vi "Osciloskop.vi"() -> ()   [LabVIEW 2023]
uses:
  <instrlib>/niScope/Controls/niScope scalar measurement.ctl
  <instrlib>/niScope/Utility/niScope Get Channel Name From String.vi
  <instrlib>/niScope/Acquire/Fetch/niScope Fetch WDT.vi
  <vilib>/express/express analysis/Spectral/Block/exnSpectralBlock spectral measurements RMS poly.vi
  <vilib>/express/express analysis/Spectral/Block/exnSpectralBlock spectral measurements RMS DDT.vi
  <vilib>/express/express analysis/Spectral/Block/exnSpectralBlock spectral measurements peak poly.vi
  <vilib>/express/express analysis/Spectral/Block/exnSpectralBlock spectral measurements peak DDT.vi
  <vilib>/express/express analysis/Spectral/Block/exnSpectralBlock spectral measurements power poly.vi
  <vilib>/express/express analysis/Spectral/Block/exnSpectralBlock spectral measurements power DDT.vi
  <vilib>/express/express analysis/Spectral/Block/exnSpectralBlock spectral measurements PSD poly.vi
  <vilib>/express/express analysis/Spectral/Block/exnSpectralBlock spectral measurements PSD DDT.vi
  <vilib>/express/express analysis/Spectral/XNode/ExpressSpectralMeasurementsBlockNode.xnode
panel:
  in  "Resource name":refnum<k15> caption="Device"
  in  "Start/Pause":bool
  in  "Simulation":bool
  in  "Measurement 5":T1=6 caption="Measurement 4" items=["None"=4000, "Frequency"=2, "Average Frequency"=1016, "FFT Frequency"=1008, "Period"=3, "Average Period"=1015, "Rise Time"=0, "Fall Time"=1, "Rising Slew Rate"=1010, "Falling Slew Rate"=1011, "Overshoot"=18, "Preshoot"=19, "Voltage RMS"=4, "Voltage Cycle RMS"=16, "AC Estimate"=1012, "FFT Amplitude"=1009, "Voltage Average"=10, "Voltage Cycle Average"=17, "DC Estimate"=1013, "Voltage Max"=6, "Voltage Min"=7, "Voltage Peak-to-Peak"=5, "Voltage High"=8, "Voltage Low"=9, "Voltage Amplitude"=15, "Voltage Top"=1007, "Voltage Base"=1006, "Voltage Base-to-Top"=1017, "Negative Width"=11, "Positive Width"=12, "Negative Duty Cycle"=13, "Positive Duty Cycle"=14, "Integral"=1005, "Area"=1003, "Cycle Area"=1004, "Time Delay"=1014, "Phase Delay"=1018, "Low Ref Volts"=1000, "Mid Ref Volts"=1001, "High Ref Volts"=1002, "Volt. Hist. Mean"=2000, "Volt. Hist. Stdev"=2001, "Volt. Hist. Median"=2003, "Volt. Hist. Mode"=2010, "Volt. Hist. Max"=2005, "Volt. Hist. Min"=2006, "Volt. Hist. Peak-to-Peak"=2002, "Volt. Hist. Mean + Stdev"=2007, "Volt. Hist. Mean + 2 Stdev"=2008, "Volt. Hist. Mean + 3 Stdev"=2009, "Volt. Hist. Hits"=2004, "Volt. Hist. New Hits"=2011, "Time Hist. Mean"=3000, "Time Hist. Stdev"=3001, "Time Hist. Median"=3003, "Time Hist. Mode"=3010, "Time Hist. Max"=3005, "Time Hist. Min"=3006, "Time Hist. Peak-to-Peak"=3002, "Time Hist. Mean + Stdev"=3007, "Time Hist. Mean + 2 Stdev"=3008, "Time Hist. Mean + 3 Stdev"=3009, "Time Hist. Hits"=3004, "Time Hist. New Hits"=3011]
  in  "Measurement 4":T1=5 caption="Measurement 3" items=["None"=4000, "Frequency"=2, "Average Frequency"=1016, "FFT Frequency"=1008, "Period"=3, "Average Period"=1015, "Rise Time"=0, "Fall Time"=1, "Rising Slew Rate"=1010, "Falling Slew Rate"=1011, "Overshoot"=18, "Preshoot"=19, "Voltage RMS"=4, "Voltage Cycle RMS"=16, "AC Estimate"=1012, "FFT Amplitude"=1009, "Voltage Average"=10, "Voltage Cycle Average"=17, "DC Estimate"=1013, "Voltage Max"=6, "Voltage Min"=7, "Voltage Peak-to-Peak"=5, "Voltage High"=8, "Voltage Low"=9, "Voltage Amplitude"=15, "Voltage Top"=1007, "Voltage Base"=1006, "Voltage Base-to-Top"=1017, "Negative Width"=11, "Positive Width"=12, "Negative Duty Cycle"=13, "Positive Duty Cycle"=14, "Integral"=1005, "Area"=1003, "Cycle Area"=1004, "Time Delay"=1014, "Phase Delay"=1018, "Low Ref Volts"=1000, "Mid Ref Volts"=1001, "High Ref Volts"=1002, "Volt. Hist. Mean"=2000, "Volt. Hist. Stdev"=2001, "Volt. Hist. Median"=2003, "Volt. Hist. Mode"=2010, "Volt. Hist. Max"=2005, "Volt. Hist. Min"=2006, "Volt. Hist. Peak-to-Peak"=2002, "Volt. Hist. Mean + Stdev"=2007, "Volt. Hist. Mean + 2 Stdev"=2008, "Volt. Hist. Mean + 3 Stdev"=2009, "Volt. Hist. Hits"=2004, "Volt. Hist. New Hits"=2011, "Time Hist. Mean"=3000, "Time Hist. Stdev"=3001, "Time Hist. Median"=3003, "Time Hist. Mode"=3010, "Time Hist. Max"=3005, "Time Hist. Min"=3006, "Time Hist. Peak-to-Peak"=3002, "Time Hist. Mean + Stdev"=3007, "Time Hist. Mean + 2 Stdev"=3008, "Time Hist. Mean + 3 Stdev"=3009, "Time Hist. Hits"=3004, "Time Hist. New Hits"=3011]
  in  "Measurement 3":T1 caption="Measurement 2" items=["None"=4000, "Frequency"=2, "Average Frequency"=1016, "FFT Frequency"=1008, "Period"=3, "Average Period"=1015, "Rise Time"=0, "Fall Time"=1, "Rising Slew Rate"=1010, "Falling Slew Rate"=1011, "Overshoot"=18, "Preshoot"=19, "Voltage RMS"=4, "Voltage Cycle RMS"=16, "AC Estimate"=1012, "FFT Amplitude"=1009, "Voltage Average"=10, "Voltage Cycle Average"=17, "DC Estimate"=1013, "Voltage Max"=6, "Voltage Min"=7, "Voltage Peak-to-Peak"=5, "Voltage High"=8, "Voltage Low"=9, "Voltage Amplitude"=15, "Voltage Top"=1007, "Voltage Base"=1006, "Voltage Base-to-Top"=1017, "Negative Width"=11, "Positive Width"=12, "Negative Duty Cycle"=13, "Positive Duty Cycle"=14, "Integral"=1005, "Area"=1003, "Cycle Area"=1004, "Time Delay"=1014, "Phase Delay"=1018, "Low Ref Volts"=1000, "Mid Ref Volts"=1001, "High Ref Volts"=1002, "Volt. Hist. Mean"=2000, "Volt. Hist. Stdev"=2001, "Volt. Hist. Median"=2003, "Volt. Hist. Mode"=2010, "Volt. Hist. Max"=2005, "Volt. Hist. Min"=2006, "Volt. Hist. Peak-to-Peak"=2002, "Volt. Hist. Mean + Stdev"=2007, "Volt. Hist. Mean + 2 Stdev"=2008, "Volt. Hist. Mean + 3 Stdev"=2009, "Volt. Hist. Hits"=2004, "Volt. Hist. New Hits"=2011, "Time Hist. Mean"=3000, "Time Hist. Stdev"=3001, "Time Hist. Median"=3003, "Time Hist. Mode"=3010, "Time Hist. Max"=3005, "Time Hist. Min"=3006, "Time Hist. Peak-to-Peak"=3002, "Time Hist. Mean + Stdev"=3007, "Time Hist. Mean + 2 Stdev"=3008, "Time Hist. Mean + 3 Stdev"=3009, "Time Hist. Hits"=3004, "Time Hist. New Hits"=3011]
  in  "Measurement 2":T1=2 caption="Measurement 1" items=["None"=4000, "Frequency"=2, "Average Frequency"=1016, "FFT Frequency"=1008, "Period"=3, "Average Period"=1015, "Rise Time"=0, "Fall Time"=1, "Rising Slew Rate"=1010, "Falling Slew Rate"=1011, "Overshoot"=18, "Preshoot"=19, "Voltage RMS"=4, "Voltage Cycle RMS"=16, "AC Estimate"=1012, "FFT Amplitude"=1009, "Voltage Average"=10, "Voltage Cycle Average"=17, "DC Estimate"=1013, "Voltage Max"=6, "Voltage Min"=7, "Voltage Peak-to-Peak"=5, "Voltage High"=8, "Voltage Low"=9, "Voltage Amplitude"=15, "Voltage Top"=1007, "Voltage Base"=1006, "Voltage Base-to-Top"=1017, "Negative Width"=11, "Positive Width"=12, "Negative Duty Cycle"=13, "Positive Duty Cycle"=14, "Integral"=1005, "Area"=1003, "Cycle Area"=1004, "Time Delay"=1014, "Phase Delay"=1018, "Low Ref Volts"=1000, "Mid Ref Volts"=1001, "High Ref Volts"=1002, "Volt. Hist. Mean"=2000, "Volt. Hist. Stdev"=2001, "Volt. Hist. Median"=2003, "Volt. Hist. Mode"=2010, "Volt. Hist. Max"=2005, "Volt. Hist. Min"=2006, "Volt. Hist. Peak-to-Peak"=2002, "Volt. Hist. Mean + Stdev"=2007, "Volt. Hist. Mean + 2 Stdev"=2008, "Volt. Hist. Mean + 3 Stdev"=2009, "Volt. Hist. Hits"=2004, "Volt. Hist. New Hits"=2011, "Time Hist. Mean"=3000, "Time Hist. Stdev"=3001, "Time Hist. Median"=3003, "Time Hist. Mode"=3010, "Time Hist. Max"=3005, "Time Hist. Min"=3006, "Time Hist. Peak-to-Peak"=3002, "Time Hist. Mean + Stdev"=3007, "Time Hist. Mean + 2 Stdev"=3008, "Time Hist. Mean + 3 Stdev"=3009, "Time Hist. Hits"=3004, "Time Hist. New Hits"=3011]
  in  "Selected Measurement":u16(ring) items=["Magnitude(RMS)", "Magnitude(Peak)", "Power spectrum", "Power spectral density"]
  in  "Left/Right":dbl(knob) scale=-100.0..100.0
  in  "Amp":dbl=1.0 min=1.0 max=1000.0
  in  "Averaging":u16(ring) items=["None", "RMS", "Peak hold"]
  in  "Window":u16(ring) items=["None", "Hanning", "Hamming", "Blackman-Harris", "Exact Blackman", "Blackman", "Flat Top", "4 Term B-Harris", "7 Term B-Harris", "Low Sidelobe"]
  in  "FFT":bool
  out "FFT Graph":dynamicdata(graph)
  in  "Upper Cut-Off":dbl=10.0 caption="Lower Cut-Off"
  in  "Zoom H":dbl(knob)=1.0 scale=0.0..10.0
  in  "Zoom V":dbl(knob)=1.0 scale=0.0..10.0
  in  "Filter":u16(ring) items=["No filter", "Low pass", "High pass", "Band pass", "Band reject", "Smoothing"]
  in  "Lower Cut-Off":dbl=0.5
  in  "Down/Up":dbl(knob) scale=-100.0..100.0
  out "M5":dbl caption="Result  4" format="%.2f"
  out "M4":dbl caption="Result  3" format="%.2f"
  out "M3":dbl caption="Result  2" format="%.2f"
  out "M2":dbl caption="Result 1" format="%.2f"
  in  "Channel/s":string="0"
  out "Waveform Graph":waveform(dbl)[](graph)
  in  "?":bool
  # "Vertical"
  # "Horizontal"
  # "Measuring"
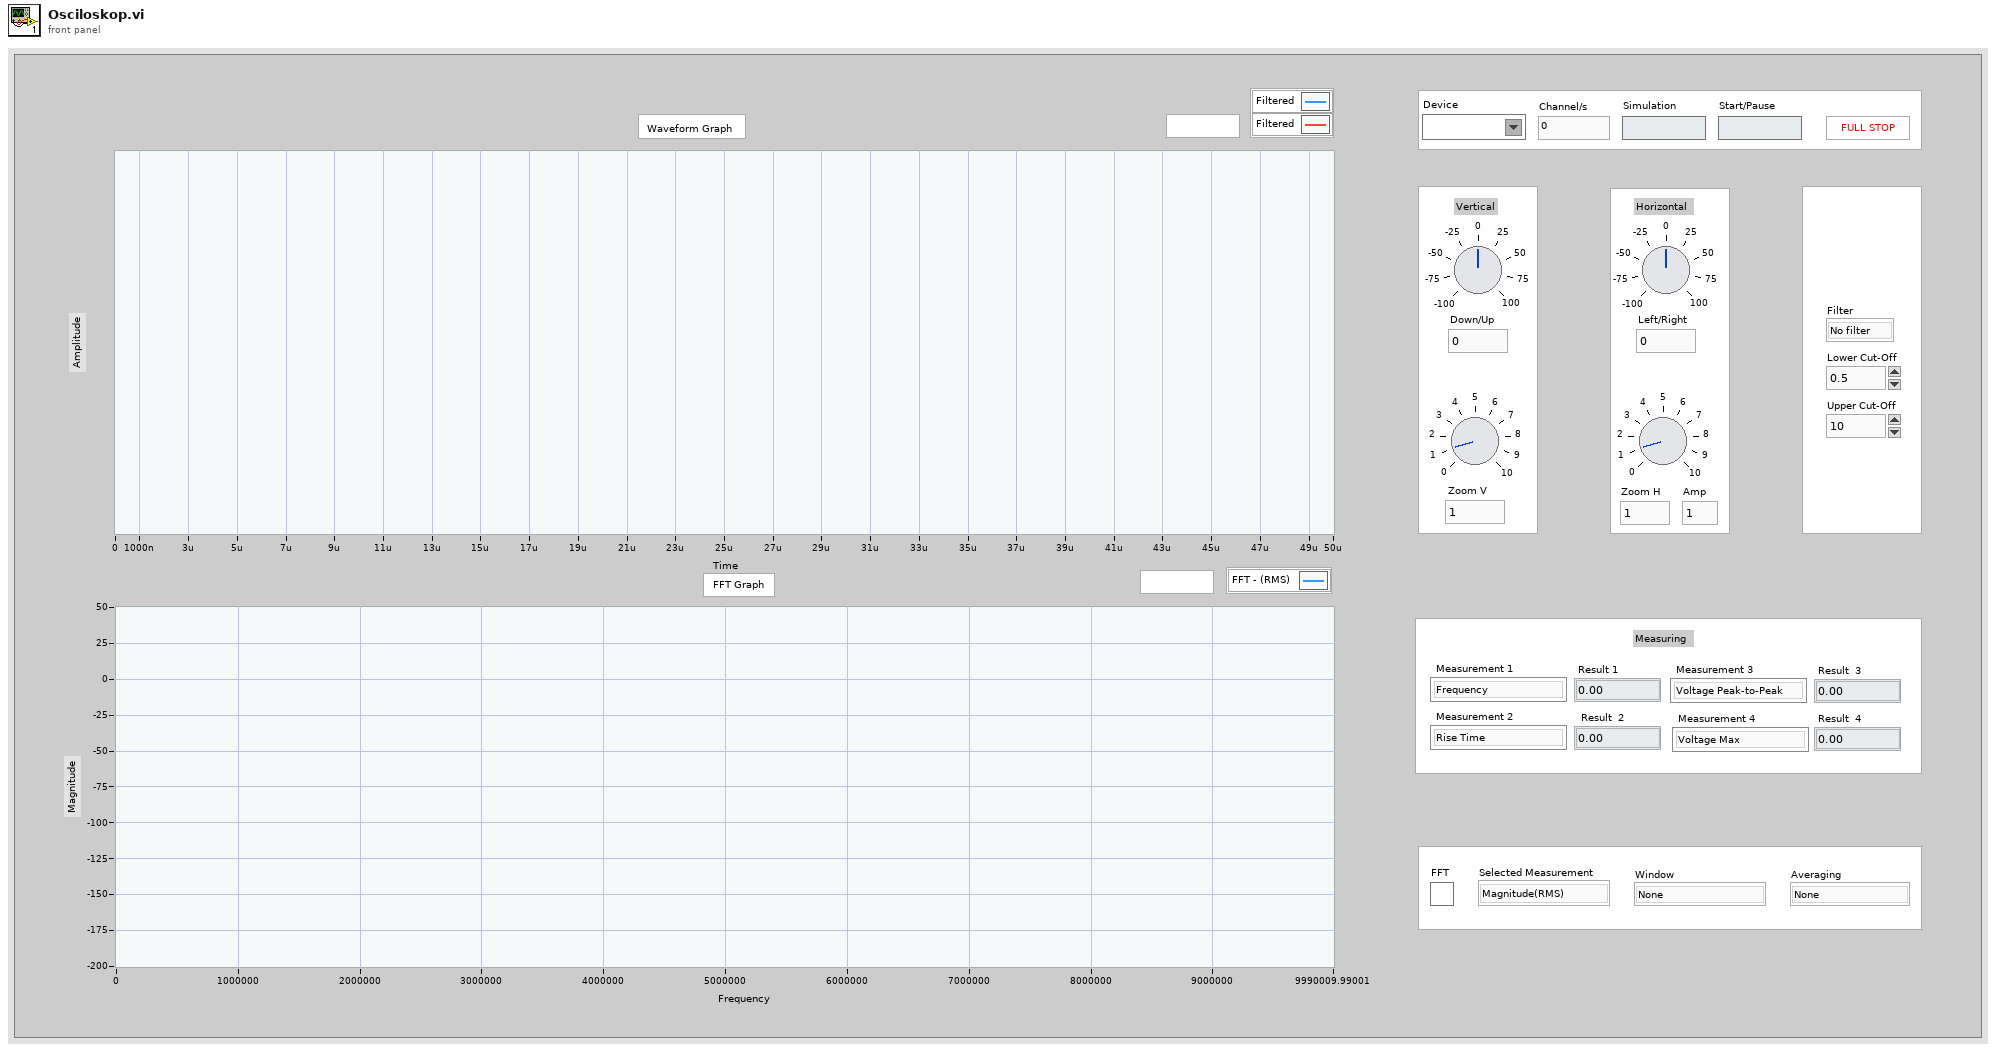
[diagram p1: front panel]
types:
  T1 = typedef "niScope scalar measurement.ctl" = i32
  T2 = cluster{"averaging mode":u16, "weighting mode":u16, "number of averages":u32}
  T3 = cluster{"dB On (F)":bool, "unwrap phase (F)":bool, "convert to degree (F)":bool}
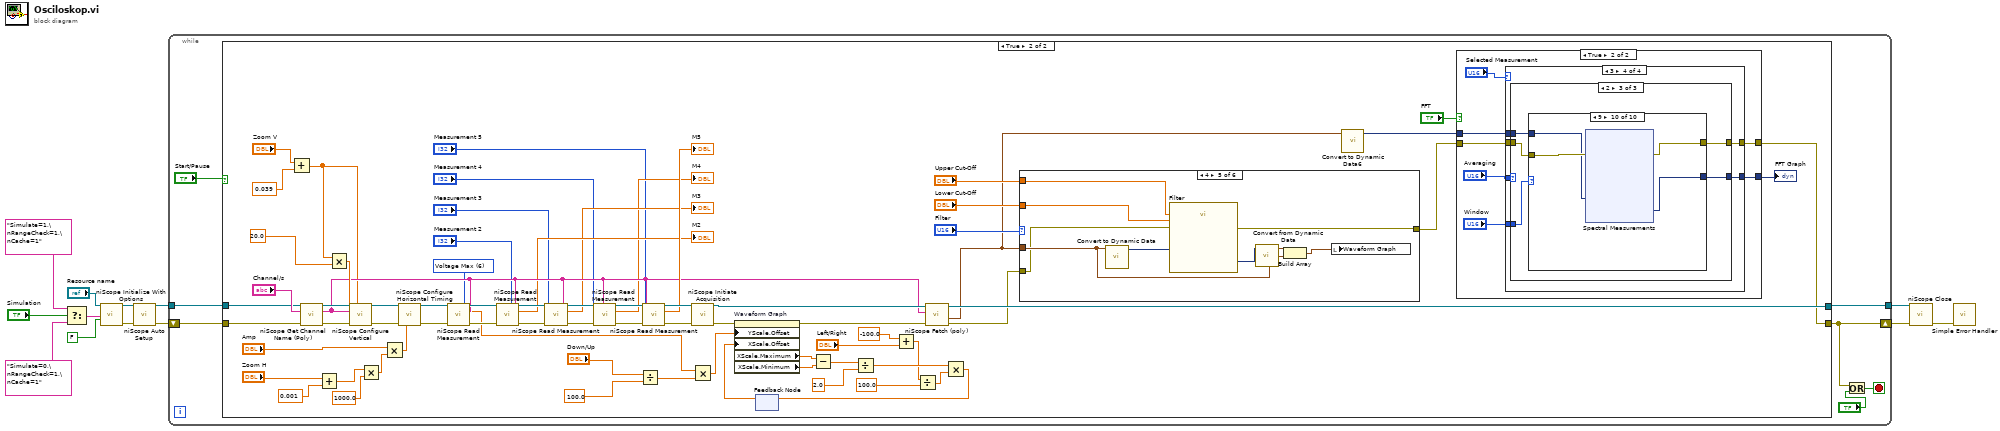
[diagram p0: block diagram]
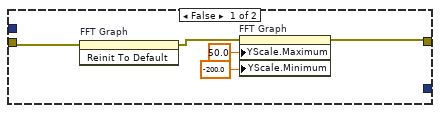
[diagram p3: hidden frame]
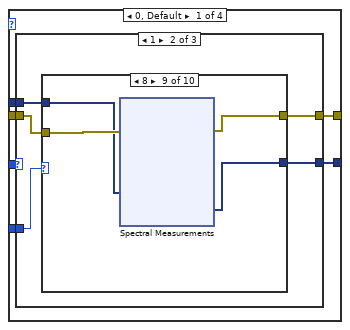
[diagram p4: hidden frame]
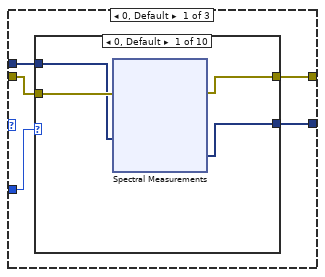
[diagram p5: hidden frame]
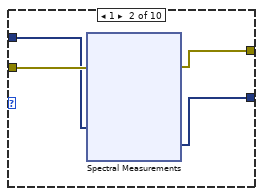
[diagram p6: hidden frame]
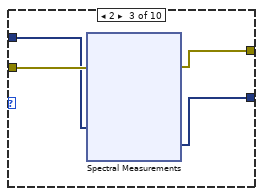
[diagram p7: hidden frame]
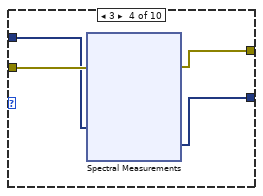
[diagram p8: hidden frame]
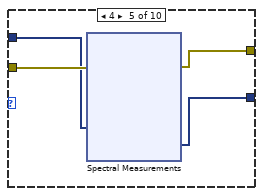
[diagram p9: hidden frame]
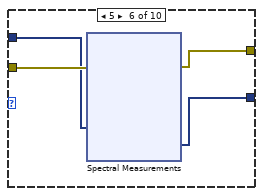
[diagram p10: hidden frame]
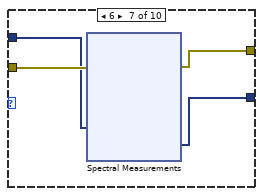
[diagram p11: hidden frame]
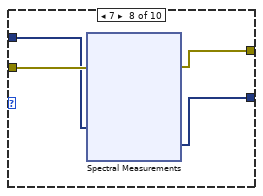
[diagram p12: hidden frame]
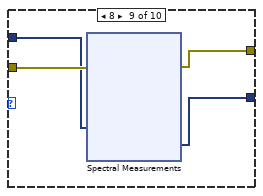
[diagram p13: hidden frame]
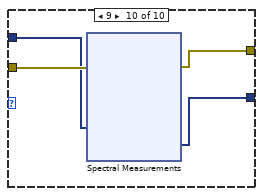
[diagram p14: hidden frame]
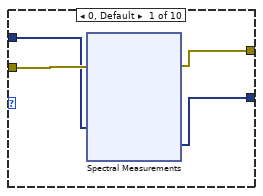
[diagram p15: hidden frame]
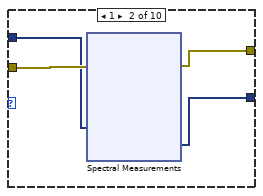
[diagram p16: hidden frame]
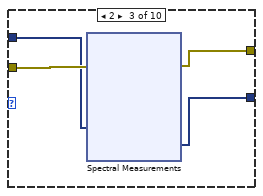
[diagram p17: hidden frame]
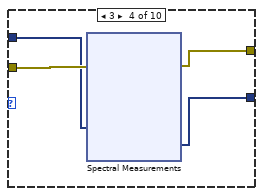
[diagram p18: hidden frame]
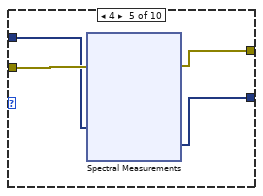
[diagram p19: hidden frame]
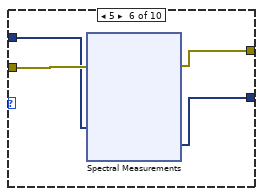
[diagram p20: hidden frame]
diagram:
  n1 = Select(t="Simulate=1,\nRangeCheck=1,\nCache=1" ("option string"), s="Simulation", f="Simulate=0,\nRangeCheck=1,\nCache=1" ("option string")) -> (s? t:f=w9:string)
  n2 = call <instrlib>:"niScope Initialize With Options.vi"("resource name"="Resource name", "option string"=w9, "reset device"=FALSE) -> ("instrument handle"=w7:refnum<k15>, "error out"=w8:errorcluster)  [unwired: 11 in]
  n3 = call <instrlib>:"niScope Auto Setup.vi"("instrument handle"=w7, "error in"=w8) -> ("instrument handle out"=w6:refnum<k15>, "error out"=w4:errorcluster)  [unwired: 12 in]
  n4 = while {
    tunnel: w6 -> [w18]
    shift-right: [w15] -> w5
    shift-left: w4 -> [w17]
    tunnel: [w16] -> w3
    stop <- w19 stop-if-true
    n5 = case shown="True" "Start/Pause" {
      tunnel: [w21 w91] -> w16
      tunnel: w17 -> [w22 w58]
      tunnel: w18 -> [w21 w57]
      tunnel: [w22 w56] -> w15
      frame False {
      }
      frame True {
        w26 = T1 6 items=["None"=4000, "Frequency"=2, "Average Frequency"=1016, "FFT Frequency"=1008, "Period"=3, "Average Period"=1015, "Rise Time"=0, "Fall Time"=1, "Rising Slew Rate"=1010, "Falling Slew Rate"=1011, "Overshoot"=18, "Preshoot"=19, "Voltage RMS"=4, "Voltage Cycle RMS"=16, "AC Estimate"=1012, "FFT Amplitude"=1009, "Voltage Average"=10, "Voltage Cycle Average"=17, "DC Estimate"=1013, "Voltage Max"=6, "Voltage Min"=7, "Voltage Peak-to-Peak"=5, "Voltage High"=8, "Voltage Low"=9, "Voltage Amplitude"=15, "Voltage Top"=1007, "Voltage Base"=1006, "Voltage Base-to-Top"=1017, "Negative Width"=11, "Positive Width"=12, "Negative Duty Cycle"=13, "Positive Duty Cycle"=14, "Integral"=1005, "Area"=1003, "Cycle Area"=1004, "Time Delay"=1014, "Phase Delay"=1018, "Low Ref Volts"=1000, "Mid Ref Volts"=1001, "High Ref Volts"=1002, "Volt. Hist. Mean"=2000, "Volt. Hist. Stdev"=2001, "Volt. Hist. Median"=2003, "Volt. Hist. Mode"=2010, "Volt. Hist. Max"=2005, "Volt. Hist. Min"=2006, "Volt. Hist. Peak-to-Peak"=2002, "Volt. Hist. Mean + Stdev"=2007, "Volt. Hist. Mean + 2 Stdev"=2008, "Volt. Hist. Mean + 3 Stdev"=2009, "Volt. Hist. Hits"=2004, "Volt. Hist. New Hits"=2011, "Time Hist. Mean"=3000, "Time Hist. Stdev"=3001, "Time Hist. Median"=3003, "Time Hist. Mode"=3010, "Time Hist. Max"=3005, "Time Hist. Min"=3006, "Time Hist. Peak-to-Peak"=3002, "Time Hist. Mean + Stdev"=3007, "Time Hist. Mean + 2 Stdev"=3008, "Time Hist. Mean + 3 Stdev"=3009, "Time Hist. Hits"=3004, "Time Hist. New Hits"=3011] ("scalar measurement")
        n6 = Add(x="Zoom V", y=0.039) -> (x+y=w23:dbl)
        n7 = call-poly <instrlib>:"niScope Get Channel Name (Poly).vi"("instrument handle"=w57, "index"="Channel/s", "error in"=w58) -> ("instrument handle out"=w94:refnum<k15>, "channel name"=w53:string, "error out"=w93:errorcluster)  [unwired: 10 in]
        n8 = Add(x="Zoom H", y=0.001) -> (x+y=w44:dbl)
        n9 = Multiply(x=w23, y=20.0) -> (x*y=w84:dbl)
        n10 = call <instrlib>:"niScope Configure Vertical.vi"("instrument handle"=w94, "probe attenuation"=w23, "channels"=w53, "vertical range"=w84, "error in"=w93) -> ("instrument handle out"=w24:refnum<k15>, "error out"=w25:errorcluster)  [unwired: 9 in]
        n11 = Multiply(x=w44, y=1000.0 ("x")) -> (x*y=w43:dbl)
        n12 = Multiply(x="Amp", y=w43) -> (x*y=w83:dbl)
        n13 = call <instrlib>:"niScope Configure Horizontal Timing.vi"("instrument handle"=w24, "error in"=w25, "min record length"=w83) -> ("instrument handle out"=w77:refnum<k15>, "error out"=w78:errorcluster)  [unwired: 11 in]
        n14 = call <instrlib>:"niScope Read Measurement.vi"("instrument handle"=w77, "channels"=w53, "scalar measurement"=w26, "error in"=w78) -> ("instrument handle out"=w68:refnum<k15>, "result"=w52:dbl, "error out"=w63:errorcluster)  [unwired: 9 in]
        n15 = call <instrlib>:"niScope Read Measurement.vi"("instrument handle"=w68, "channels"=w53, "scalar measurement"="Measurement 2", "error in"=w63) -> ("instrument handle out"=w67:refnum<k15>, "result"=→"M2":dbl, "error out"=w62:errorcluster)  [unwired: 9 in]
        n16 = call <instrlib>:"niScope Read Measurement.vi"("instrument handle"=w67, "channels"=w53, "scalar measurement"="Measurement 3", "error in"=w62) -> ("instrument handle out"=w66:refnum<k15>, "result"=→"M3":dbl, "error out"=w61:errorcluster)  [unwired: 9 in]
        n17 = call <instrlib>:"niScope Read Measurement.vi"("instrument handle"=w66, "channels"=w53, "scalar measurement"="Measurement 4", "error in"=w61) -> ("instrument handle out"=w65:refnum<k15>, "result"=→"M4":dbl, "error out"=w60:errorcluster)  [unwired: 9 in]
        n18 = Divide(x="Down/Up", y=100.0) -> (x/y=w38:dbl)
        n19 = call <instrlib>:"niScope Read Measurement.vi"("instrument handle"=w65, "channels"=w53, "scalar measurement"="Measurement 5", "error in"=w60) -> ("instrument handle out"=w64:refnum<k15>, "result"=→"M5":dbl, "error out"=w59:errorcluster)  [unwired: 9 in]
        n20 = call <instrlib>:"niScope Initiate Acquisition.vi"("instrument handle"=w64, "error in"=w59) -> ("instrument handle out"=w80:refnum<k15>, "error out"=w79:errorcluster)  [unwired: 12 in]
        n21 = Multiply(x=w52, y=w38) -> (x*y=w76:dbl)
        n22 = feedback #1() -> (w71:dbl)  [unwired: 1 in]
        n23 = property on="Waveform Graph" class="WFGraph (strict)"(error in=w79, "YScale.Offset"=w76, "XScale.Offset"=w71) -> (error out=w82:errorcluster, "XScale.Maximum"=w36:dbl, "XScale.Minimum"=w35:dbl)  [unwired: 1 in, 1 out]
        n24 = Subtract(x=w36, y=w35) -> (x-y=w75:dbl)
        n25 = Divide(x=w75, y=2.0) -> (x/y=w73:dbl)
        n26 = Add(x=-100.0, y="Left/Right") -> (x+y=w33:dbl)
        n27 = Divide(x=w33, y=100.0) -> (x/y=w32:dbl)
        n28 = call-poly <instrlib>:"niScope Fetch (poly).vi"("error in"=w82, "channels"=w53, "instrument handle"=w80) -> ("error out"=w27:errorcluster, "wfm"=w28:waveform(dbl), "instrument handle out"=w91:refnum<k15>)  [unwired: 5 in, 1 out]
        n29 = Multiply(x=w73, y=w32) -> (x*y=w72:dbl)
        n30 = feedback-in #1(w72) -> ()
        n31 = case shown="4" "Filter" {
          tunnel: "Lower Cut-Off" -> [_ w1900 w1908 w1918 w1927 _]
          tunnel: w28 -> [w1893 w1897 w1905 w1914 w1923 w1932]
          tunnel: "Upper Cut-Off" -> [_ _ _ w1912 w1921 _]
          tunnel: w27 -> [w1891 w1895 w1903 w1910 w1920 w1928]
          tunnel: [w1891 w1894 w1902 w1911 w1919 w1929] -> w55
          frame 0, Default {
            n32 = Build Array(w1893, w1893) -> (→"Waveform Graph":waveform(dbl)[])
          }
          frame 1 {
            n33 = call "Convert to Dynamic Data2"("Waveform"=w1897) -> ("Dynamic Data Type"=w1899:dynamicdata)  [unwired: 3 in]
            n34 = call "Filter2"("error in (no error)"=w1895, "Lower Cut-Off"=w1900, "Signal"=w1899) -> ("error out"=w1894:errorcluster, "Filtered Signal"=w1901:dynamicdata)  [unwired: 7 in]
            n35 = call "Convert from Dynamic Data2"("Dynamic Data Type"=w1901) -> ("Waveform"=w1898:waveform(dbl))  [unwired: 3 in]
            n36 = Build Array(w1898, w1897) -> (w1896:waveform(dbl)[])
            n37 = local write "Waveform Graph"(w1896) -> ()
          }
          frame 2 {
            n38 = call "Convert to Dynamic Data3"("Waveform"=w1905) -> ("Dynamic Data Type"=w1907:dynamicdata)  [unwired: 3 in]
            n39 = call "Filter3"("error in (no error)"=w1903, "Lower Cut-Off"=w1908, "Signal"=w1907) -> ("error out"=w1902:errorcluster, "Filtered Signal"=w1909:dynamicdata)  [unwired: 7 in]
            n40 = call "Convert from Dynamic Data3"("Dynamic Data Type"=w1909) -> ("Waveform"=w1906:waveform(dbl))  [unwired: 3 in]
            n41 = Build Array(w1906, w1905) -> (w1904:waveform(dbl)[])
            n42 = local write "Waveform Graph"(w1904) -> ()
          }
          frame 3 {
            n43 = call "Convert to Dynamic Data4"("Waveform"=w1914) -> ("Dynamic Data Type"=w1917:dynamicdata)  [unwired: 3 in]
            n44 = call "Filter4"("error in (no error)"=w1910, "Lower Cut-Off"=w1918, "Upper Cut-Off"=w1912, "Signal"=w1917) -> ("error out"=w1911:errorcluster, "Filtered Signal"=w1916:dynamicdata)  [unwired: 6 in]
            n45 = call "Convert from Dynamic Data4"("Dynamic Data Type"=w1916, "Channel"=w1916) -> ("Waveform"=w1915:waveform(dbl))  [unwired: 2 in]
            n46 = Build Array(w1915, w1914) -> (w1913:waveform(dbl)[])
            n47 = local write "Waveform Graph"(w1913) -> ()
          }
          frame 4 {
            n48 = call "Convert to Dynamic Data"("Waveform"=w1923) -> ("Dynamic Data Type"=w1926:dynamicdata)  [unwired: 3 in]
            n49 = call "Filter"("error in (no error)"=w1920, "Lower Cut-Off"=w1927, "Upper Cut-Off"=w1921, "Signal"=w1926) -> ("error out"=w1919:errorcluster, "Filtered Signal"=w1925:dynamicdata)  [unwired: 6 in]
            n50 = call "Convert from Dynamic Data"("Dynamic Data Type"=w1925, "Channel"=w1925) -> ("Waveform"=w1924:waveform(dbl))  [unwired: 2 in]
            n51 = Build Array(w1924, w1923) -> (w1922:waveform(dbl)[])
            n52 = local write "Waveform Graph"(w1922) -> ()
          }
          frame 5 {
            n53 = call "Convert to Dynamic Data5"("Waveform"=w1932) -> ("Dynamic Data Type"=w1934:dynamicdata)  [unwired: 3 in]
            n54 = call "Filter5"("error in (no error)"=w1928, "Signal"=w1934) -> ("error out"=w1929:errorcluster, "Filtered Signal"=w1933:dynamicdata)  [unwired: 8 in]
            n55 = call "Convert from Dynamic Data5"("Dynamic Data Type"=w1933, "Channel"=w1933) -> ("Waveform"=w1930:waveform(dbl))  [unwired: 2 in]
            n56 = Build Array(w1930, w1930) -> (w1931:waveform(dbl)[])
            n57 = local write "Waveform Graph"(w1931) -> ()
          }
        }
        n58 = call "Convert to Dynamic Data6"("Waveform"=w28) -> ("Dynamic Data Type"=w86:dynamicdata)  [unwired: 3 in]
        n59 = case shown="True" "FFT" {
          tunnel: w55 -> [w99 w104]
          tunnel: [w97 w102] -> w56
          tunnel: w86 -> [_ w103]
          tunnel: [_ w100] -> w85
          frame False {
            n60 = invoke on="FFT Graph" class="WFGraph (strict)" method="Reinit To Default"(error in=w99) -> (error out=w98:errorcluster)  [unwired: 2 in, 2 out]
            n61 = property on="FFT Graph" class="WFGraph (strict)"(error in=w98, "YScale.Maximum"=50.0 ("Y Scale.Range:Maximum"), "YScale.Minimum"=-200.0 ("Y Scale.Range:Minimum")) -> (error out=w97:errorcluster)  [unwired: 1 in, 1 out]
          }
          frame True {
            n62 = case shown="3" "Selected Measurement" {
              tunnel: "Averaging" -> [w112 w573 w1034 w1465]
              tunnel: "Window" -> [w111 w572 w1033 w1464]
              tunnel: w104 -> [w110 w571 w1032 w1463]
              tunnel: w103 -> [w109 w570 w1031 w1462]
              tunnel: [w108 w569 w1030 w1461] -> w102
              tunnel: [w107 w568 w1029 w1460] -> w100
              frame 0, Default {
                n63 = case shown="1" w112 {
                  tunnel: w111 -> [w117 w262 w417]
                  tunnel: w110 -> [w116 w261 w416]
                  tunnel: w109 -> [w115 w260 w415]
                  tunnel: [w114 w259 w414] -> w108
                  tunnel: [w113 w258 w413] -> w107
                  frame 0, Default {
                    n64 = case shown="0, Default" w117 {
                      tunnel: w116 -> [w121 w135 w149 w163 w177 w191 w205 w219 w233 w247]
                      tunnel: w115 -> [w120 w134 w148 w162 w176 w190 w204 w218 w232 w246]
                      tunnel: [w119 w133 w147 w161 w175 w189 w203 w217 w231 w245] -> w114
                      tunnel: [w118 w132 w146 w160 w174 w188 w202 w216 w230 w244] -> w113
                      frame 0, Default {
                        n65 = xnode "Spectral Measurements"("Signals"=w120, "error in (no error)"=w121) -> ("FFT - (RMS)"=w118:dynamicdata, "error out"=w119:errorcluster)  [unwired: 1 out]
                      }
                      frame 1 {
                        n66 = xnode "Spectral Measurements"("Signals"=w134, "error in (no error)"=w135) -> ("FFT - (RMS)"=w132:dynamicdata, "error out"=w133:errorcluster)  [unwired: 1 out]
                      }
                      frame 2 {
                        n67 = xnode "Spectral Measurements"("Signals"=w148, "error in (no error)"=w149) -> ("FFT - (RMS)"=w146:dynamicdata, "error out"=w147:errorcluster)  [unwired: 1 out]
                      }
                      frame 3 {
                        n68 = xnode "Spectral Measurements"("Signals"=w162, "error in (no error)"=w163) -> ("FFT - (RMS)"=w160:dynamicdata, "error out"=w161:errorcluster)  [unwired: 1 out]
                      }
                      frame 4 {
                        n69 = xnode "Spectral Measurements"("Signals"=w176, "error in (no error)"=w177) -> ("FFT - (RMS)"=w174:dynamicdata, "error out"=w175:errorcluster)  [unwired: 1 out]
                      }
                      frame 5 {
                        n70 = xnode "Spectral Measurements"("Signals"=w190, "error in (no error)"=w191) -> ("FFT - (RMS)"=w188:dynamicdata, "error out"=w189:errorcluster)  [unwired: 1 out]
                      }
                      frame 6 {
                        n71 = xnode "Spectral Measurements"("Signals"=w204, "error in (no error)"=w205) -> ("FFT - (RMS)"=w202:dynamicdata, "error out"=w203:errorcluster)  [unwired: 1 out]
                      }
                      frame 7 {
                        n72 = xnode "Spectral Measurements"("Signals"=w218, "error in (no error)"=w219) -> ("FFT - (RMS)"=w216:dynamicdata, "error out"=w217:errorcluster)  [unwired: 1 out]
                      }
                      frame 8 {
                        n73 = xnode "Spectral Measurements"("Signals"=w232, "error in (no error)"=w233) -> ("FFT - (RMS)"=w230:dynamicdata, "error out"=w231:errorcluster)  [unwired: 1 out]
                      }
                      frame 9 {
                        n74 = xnode "Spectral Measurements"("Signals"=w246, "error in (no error)"=w247) -> ("FFT - (RMS)"=w244:dynamicdata, "error out"=w245:errorcluster)  [unwired: 1 out]
                      }
                    }
                  }
                  frame 1 {
                    n75 = case shown="8" w262 {
                      tunnel: w261 -> [w266 w281 w296 w311 w326 w341 w356 w371 w386 w401]
                      tunnel: w260 -> [w265 w280 w295 w310 w325 w340 w355 w370 w385 w400]
                      tunnel: [w264 w279 w294 w309 w324 w339 w354 w369 w384 w399] -> w259
                      tunnel: [w263 w278 w293 w308 w323 w338 w353 w368 w383 w398] -> w258
                      frame 0, Default {
                        n76 = xnode "Spectral Measurements"("Signals"=w265, "error in (no error)"=w266) -> ("FFT - (RMS)"=w263:dynamicdata, "error out"=w264:errorcluster)  [unwired: 1 in, 2 out]
                      }
                      frame 1 {
                        n77 = xnode "Spectral Measurements"("Signals"=w280, "error in (no error)"=w281) -> ("FFT - (RMS)"=w278:dynamicdata, "error out"=w279:errorcluster)  [unwired: 1 in, 2 out]
                      }
                      frame 2 {
                        n78 = xnode "Spectral Measurements"("Signals"=w295, "error in (no error)"=w296) -> ("FFT - (RMS)"=w293:dynamicdata, "error out"=w294:errorcluster)  [unwired: 1 in, 2 out]
                      }
                      frame 3 {
                        n79 = xnode "Spectral Measurements"("Signals"=w310, "error in (no error)"=w311) -> ("FFT - (RMS)"=w308:dynamicdata, "error out"=w309:errorcluster)  [unwired: 1 in, 2 out]
                      }
                      frame 4 {
                        n80 = xnode "Spectral Measurements"("Signals"=w325, "error in (no error)"=w326) -> ("FFT - (RMS)"=w323:dynamicdata, "error out"=w324:errorcluster)  [unwired: 1 in, 2 out]
                      }
                      frame 5 {
                        n81 = xnode "Spectral Measurements"("Signals"=w340, "error in (no error)"=w341) -> ("FFT - (RMS)"=w338:dynamicdata, "error out"=w339:errorcluster)  [unwired: 1 in, 2 out]
                      }
                      frame 6 {
                        n82 = xnode "Spectral Measurements"("Signals"=w355, "error in (no error)"=w356) -> ("FFT - (RMS)"=w353:dynamicdata, "error out"=w354:errorcluster)  [unwired: 1 in, 2 out]
                      }
                      frame 7 {
                        n83 = xnode "Spectral Measurements"("Signals"=w370, "error in (no error)"=w371) -> ("FFT - (RMS)"=w368:dynamicdata, "error out"=w369:errorcluster)  [unwired: 1 in, 2 out]
                      }
                      frame 8 {
                        n84 = xnode "Spectral Measurements"("Signals"=w385, "error in (no error)"=w386) -> ("FFT - (RMS)"=w383:dynamicdata, "error out"=w384:errorcluster)  [unwired: 1 in, 2 out]
                      }
                      frame 9 {
                        n85 = xnode "Spectral Measurements"("Signals"=w400, "error in (no error)"=w401) -> ("FFT - (RMS)"=w398:dynamicdata, "error out"=w399:errorcluster)  [unwired: 1 in, 2 out]
                      }
                    }
                  }
                  frame 2 {
                    n86 = case shown="9" w417 {
                      tunnel: w416 -> [w421 w436 w451 w466 w481 w496 w511 w526 w541 w556]
                      tunnel: w415 -> [w420 w435 w450 w465 w480 w495 w510 w525 w540 w555]
                      tunnel: [w419 w434 w449 w464 w479 w494 w509 w524 w539 w554] -> w414
                      tunnel: [w418 w433 w448 w463 w478 w493 w508 w523 w538 w553] -> w413
                      frame 0, Default {
                        n87 = xnode "Spectral Measurements"("Signals"=w420, "error in (no error)"=w421) -> ("FFT - (RMS)"=w418:dynamicdata, "error out"=w419:errorcluster)  [unwired: 1 in, 2 out]
                      }
                      frame 1 {
                        n88 = xnode "Spectral Measurements"("Signals"=w435, "error in (no error)"=w436) -> ("FFT - (RMS)"=w433:dynamicdata, "error out"=w434:errorcluster)  [unwired: 1 in, 2 out]
                      }
                      frame 2 {
                        n89 = xnode "Spectral Measurements"("Signals"=w450, "error in (no error)"=w451) -> ("FFT - (RMS)"=w448:dynamicdata, "error out"=w449:errorcluster)  [unwired: 1 in, 2 out]
                      }
                      frame 3 {
                        n90 = xnode "Spectral Measurements"("Signals"=w465, "error in (no error)"=w466) -> ("FFT - (RMS)"=w463:dynamicdata, "error out"=w464:errorcluster)  [unwired: 1 in, 2 out]
                      }
                      frame 4 {
                        n91 = xnode "Spectral Measurements"("Signals"=w480, "error in (no error)"=w481) -> ("FFT - (RMS)"=w478:dynamicdata, "error out"=w479:errorcluster)  [unwired: 1 in, 2 out]
                      }
                      frame 5 {
                        n92 = xnode "Spectral Measurements"("Signals"=w495, "error in (no error)"=w496) -> ("FFT - (RMS)"=w493:dynamicdata, "error out"=w494:errorcluster)  [unwired: 1 in, 2 out]
                      }
                      frame 6 {
                        n93 = xnode "Spectral Measurements"("Signals"=w510, "error in (no error)"=w511) -> ("FFT - (RMS)"=w508:dynamicdata, "error out"=w509:errorcluster)  [unwired: 1 in, 2 out]
                      }
                      frame 7 {
                        n94 = xnode "Spectral Measurements"("Signals"=w525, "error in (no error)"=w526) -> ("FFT - (RMS)"=w523:dynamicdata, "error out"=w524:errorcluster)  [unwired: 1 in, 2 out]
                      }
                      frame 8 {
                        n95 = xnode "Spectral Measurements"("Signals"=w540, "error in (no error)"=w541) -> ("FFT - (RMS)"=w538:dynamicdata, "error out"=w539:errorcluster)  [unwired: 1 in, 2 out]
                      }
                      frame 9 {
                        n96 = xnode "Spectral Measurements"("Signals"=w555, "error in (no error)"=w556) -> ("FFT - (RMS)"=w553:dynamicdata, "error out"=w554:errorcluster)  [unwired: 1 in, 2 out]
                      }
                    }
                  }
                }
              }
              frame 1 {
                n97 = case shown="2" w573 {
                  tunnel: w572 -> [w578 w723 w878]
                  tunnel: w571 -> [w577 w722 w877]
                  tunnel: w570 -> [w576 w721 w876]
                  tunnel: [w575 w720 w875] -> w569
                  tunnel: [w574 w719 w874] -> w568
                  frame 0, Default {
                    n98 = case shown="9" w578 {
                      tunnel: w577 -> [w582 w596 w610 w624 w638 w652 w666 w680 w694 w708]
                      tunnel: w576 -> [w581 w595 w609 w623 w637 w651 w665 w679 w693 w707]
                      tunnel: [w580 w594 w608 w622 w636 w650 w664 w678 w692 w706] -> w575
                      tunnel: [w579 w593 w607 w621 w635 w649 w663 w677 w691 w705] -> w574
                      frame 0, Default {
                        n99 = xnode "Spectral Measurements"("Signals"=w581, "error in (no error)"=w582) -> ("FFT - (Peak)"=w579:dynamicdata, "error out"=w580:errorcluster)  [unwired: 1 out]
                      }
                      frame 1 {
                        n100 = xnode "Spectral Measurements"("Signals"=w595, "error in (no error)"=w596) -> ("FFT - (Peak)"=w593:dynamicdata, "error out"=w594:errorcluster)  [unwired: 1 out]
                      }
                      frame 2 {
                        n101 = xnode "Spectral Measurements"("Signals"=w609, "error in (no error)"=w610) -> ("FFT - (Peak)"=w607:dynamicdata, "error out"=w608:errorcluster)  [unwired: 1 out]
                      }
                      frame 3 {
                        n102 = xnode "Spectral Measurements"("Signals"=w623, "error in (no error)"=w624) -> ("FFT - (Peak)"=w621:dynamicdata, "error out"=w622:errorcluster)  [unwired: 1 out]
                      }
                      frame 4 {
                        n103 = xnode "Spectral Measurements"("Signals"=w637, "error in (no error)"=w638) -> ("FFT - (Peak)"=w635:dynamicdata, "error out"=w636:errorcluster)  [unwired: 1 out]
                      }
                      frame 5 {
                        n104 = xnode "Spectral Measurements"("Signals"=w651, "error in (no error)"=w652) -> ("FFT - (Peak)"=w649:dynamicdata, "error out"=w650:errorcluster)  [unwired: 1 out]
                      }
                      frame 6 {
                        n105 = xnode "Spectral Measurements"("Signals"=w665, "error in (no error)"=w666) -> ("FFT - (Peak)"=w663:dynamicdata, "error out"=w664:errorcluster)  [unwired: 1 out]
                      }
                      frame 7 {
                        n106 = xnode "Spectral Measurements"("Signals"=w679, "error in (no error)"=w680) -> ("FFT - (Peak)"=w677:dynamicdata, "error out"=w678:errorcluster)  [unwired: 1 out]
                      }
                      frame 8 {
                        n107 = xnode "Spectral Measurements"("Signals"=w693, "error in (no error)"=w694) -> ("FFT - (Peak)"=w691:dynamicdata, "error out"=w692:errorcluster)  [unwired: 1 out]
                      }
                      frame 9 {
                        n108 = xnode "Spectral Measurements"("Signals"=w707, "error in (no error)"=w708) -> ("FFT - (Peak)"=w705:dynamicdata, "error out"=w706:errorcluster)  [unwired: 1 out]
                      }
                    }
                  }
                  frame 1 {
                    n109 = case shown="9" w723 {
                      tunnel: w722 -> [w727 w742 w757 w772 w787 w802 w817 w832 w847 w862]
                      tunnel: w721 -> [w726 w741 w756 w771 w786 w801 w816 w831 w846 w861]
                      tunnel: [w725 w740 w755 w770 w785 w800 w815 w830 w845 w860] -> w720
                      tunnel: [w724 w739 w754 w769 w784 w799 w814 w829 w844 w859] -> w719
                      frame 0, Default {
                        n110 = xnode "Spectral Measurements"("Signals"=w726, "error in (no error)"=w727) -> ("FFT - (Peak)"=w724:dynamicdata, "error out"=w725:errorcluster)  [unwired: 1 in, 2 out]
                      }
                      frame 1 {
                        n111 = xnode "Spectral Measurements"("Signals"=w741, "error in (no error)"=w742) -> ("FFT - (Peak)"=w739:dynamicdata, "error out"=w740:errorcluster)  [unwired: 1 in, 2 out]
                      }
                      frame 2 {
                        n112 = xnode "Spectral Measurements"("Signals"=w756, "error in (no error)"=w757) -> ("FFT - (Peak)"=w754:dynamicdata, "error out"=w755:errorcluster)  [unwired: 1 in, 2 out]
                      }
                      frame 3 {
                        n113 = xnode "Spectral Measurements"("Signals"=w771, "error in (no error)"=w772) -> ("FFT - (Peak)"=w769:dynamicdata, "error out"=w770:errorcluster)  [unwired: 1 in, 2 out]
                      }
                      frame 4 {
                        n114 = xnode "Spectral Measurements"("Signals"=w786, "error in (no error)"=w787) -> ("FFT - (Peak)"=w784:dynamicdata, "error out"=w785:errorcluster)  [unwired: 1 in, 2 out]
                      }
                      frame 5 {
                        n115 = xnode "Spectral Measurements"("Signals"=w801, "error in (no error)"=w802) -> ("FFT - (Peak)"=w799:dynamicdata, "error out"=w800:errorcluster)  [unwired: 1 in, 2 out]
                      }
                      frame 6 {
                        n116 = xnode "Spectral Measurements"("Signals"=w816, "error in (no error)"=w817) -> ("FFT - (Peak)"=w814:dynamicdata, "error out"=w815:errorcluster)  [unwired: 1 in, 2 out]
                      }
                      frame 7 {
                        n117 = xnode "Spectral Measurements"("Signals"=w831, "error in (no error)"=w832) -> ("FFT - (Peak)"=w829:dynamicdata, "error out"=w830:errorcluster)  [unwired: 1 in, 2 out]
                      }
                      frame 8 {
                        n118 = xnode "Spectral Measurements"("Signals"=w846, "error in (no error)"=w847) -> ("FFT - (Peak)"=w844:dynamicdata, "error out"=w845:errorcluster)  [unwired: 1 in, 2 out]
                      }
                      frame 9 {
                        n119 = xnode "Spectral Measurements"("Signals"=w861, "error in (no error)"=w862) -> ("FFT - (Peak)"=w859:dynamicdata, "error out"=w860:errorcluster)  [unwired: 1 in, 2 out]
                      }
                    }
                  }
                  frame 2 {
                    n120 = case shown="5" w878 {
                      tunnel: w877 -> [w882 w897 w912 w927 w942 w957 w972 w987 w1002 w1017]
                      tunnel: w876 -> [w881 w896 w911 w926 w941 w956 w971 w986 w1001 w1016]
                      tunnel: [w880 w895 w910 w925 w940 w955 w970 w985 w1000 w1015] -> w875
                      tunnel: [w879 w894 w909 w924 w939 w954 w969 w984 w999 w1014] -> w874
                      frame 0, Default {
                        n121 = xnode "Spectral Measurements"("Signals"=w881, "error in (no error)"=w882) -> ("FFT - (Peak)"=w879:dynamicdata, "error out"=w880:errorcluster)  [unwired: 1 in, 2 out]
                      }
                      frame 1 {
                        n122 = xnode "Spectral Measurements"("Signals"=w896, "error in (no error)"=w897) -> ("FFT - (Peak)"=w894:dynamicdata, "error out"=w895:errorcluster)  [unwired: 1 in, 2 out]
                      }
                      frame 2 {
                        n123 = xnode "Spectral Measurements"("Signals"=w911, "error in (no error)"=w912) -> ("FFT - (Peak)"=w909:dynamicdata, "error out"=w910:errorcluster)  [unwired: 1 in, 2 out]
                      }
                      frame 3 {
                        n124 = xnode "Spectral Measurements"("Signals"=w926, "error in (no error)"=w927) -> ("FFT - (Peak)"=w924:dynamicdata, "error out"=w925:errorcluster)  [unwired: 1 in, 2 out]
                      }
                      frame 4 {
                        n125 = xnode "Spectral Measurements"("Signals"=w941, "error in (no error)"=w942) -> ("FFT - (Peak)"=w939:dynamicdata, "error out"=w940:errorcluster)  [unwired: 1 in, 2 out]
                      }
                      frame 5 {
                        n126 = xnode "Spectral Measurements"("Signals"=w956, "error in (no error)"=w957) -> ("FFT - (Peak)"=w954:dynamicdata, "error out"=w955:errorcluster)  [unwired: 1 in, 2 out]
                      }
                      frame 6 {
                        n127 = xnode "Spectral Measurements"("Signals"=w971, "error in (no error)"=w972) -> ("FFT - (Peak)"=w969:dynamicdata, "error out"=w970:errorcluster)  [unwired: 1 in, 2 out]
                      }
                      frame 7 {
                        n128 = xnode "Spectral Measurements"("Signals"=w986, "error in (no error)"=w987) -> ("FFT - (Peak)"=w984:dynamicdata, "error out"=w985:errorcluster)  [unwired: 1 in, 2 out]
                      }
                      frame 8 {
                        n129 = xnode "Spectral Measurements"("Signals"=w1001, "error in (no error)"=w1002) -> ("FFT - (Peak)"=w999:dynamicdata, "error out"=w1000:errorcluster)  [unwired: 1 in, 2 out]
                      }
                      frame 9 {
                        n130 = xnode "Spectral Measurements"("Signals"=w1016, "error in (no error)"=w1017) -> ("FFT - (Peak)"=w1014:dynamicdata, "error out"=w1015:errorcluster)  [unwired: 1 in, 2 out]
                      }
                    }
                  }
                }
              }
              frame 2 {
                n131 = case shown="0, Default" w1034 {
                  tunnel: w1033 -> [w1039 w1174 w1319]
                  tunnel: w1032 -> [w1038 w1173 w1318]
                  tunnel: w1031 -> [w1037 w1172 w1317]
                  tunnel: [w1036 w1171 w1316] -> w1030
                  tunnel: [w1035 w1170 w1315] -> w1029
                  frame 0, Default {
                    n132 = case shown="6" w1039 {
                      tunnel: w1038 -> [w1043 w1056 w1069 w1082 w1095 w1108 w1121 w1134 w1147 w1160]
                      tunnel: w1037 -> [w1042 w1055 w1068 w1081 w1094 w1107 w1120 w1133 w1146 w1159]
                      tunnel: [w1041 w1054 w1067 w1080 w1093 w1106 w1119 w1132 w1145 w1158] -> w1036
                      tunnel: [w1040 w1053 w1066 w1079 w1092 w1105 w1118 w1131 w1144 w1157] -> w1035
                      frame 0, Default {
                        n133 = xnode "Spectral Measurements"("Signals"=w1042, "error in (no error)"=w1043) -> ("Power Spectrum"=w1040:dynamicdata, "error out"=w1041:errorcluster)
                      }
                      frame 1 {
                        n134 = xnode "Spectral Measurements"("Signals"=w1055, "error in (no error)"=w1056) -> ("Power Spectrum"=w1053:dynamicdata, "error out"=w1054:errorcluster)
                      }
                      frame 2 {
                        n135 = xnode "Spectral Measurements"("Signals"=w1068, "error in (no error)"=w1069) -> ("Power Spectrum"=w1066:dynamicdata, "error out"=w1067:errorcluster)
                      }
                      frame 3 {
                        n136 = xnode "Spectral Measurements"("Signals"=w1081, "error in (no error)"=w1082) -> ("Power Spectrum"=w1079:dynamicdata, "error out"=w1080:errorcluster)
                      }
                      frame 4 {
                        n137 = xnode "Spectral Measurements"("Signals"=w1094, "error in (no error)"=w1095) -> ("Power Spectrum"=w1092:dynamicdata, "error out"=w1093:errorcluster)
                      }
                      frame 5 {
                        n138 = xnode "Spectral Measurements"("Signals"=w1107, "error in (no error)"=w1108) -> ("Power Spectrum"=w1105:dynamicdata, "error out"=w1106:errorcluster)
                      }
                      frame 6 {
                        n139 = xnode "Spectral Measurements"("Signals"=w1120, "error in (no error)"=w1121) -> ("Power Spectrum"=w1118:dynamicdata, "error out"=w1119:errorcluster)
                      }
                      frame 7 {
                        n140 = xnode "Spectral Measurements"("Signals"=w1133, "error in (no error)"=w1134) -> ("Power Spectrum"=w1131:dynamicdata, "error out"=w1132:errorcluster)
                      }
                      frame 8 {
                        n141 = xnode "Spectral Measurements"("Signals"=w1146, "error in (no error)"=w1147) -> ("Power Spectrum"=w1144:dynamicdata, "error out"=w1145:errorcluster)
                      }
                      frame 9 {
                        n142 = xnode "Spectral Measurements"("Signals"=w1159, "error in (no error)"=w1160) -> ("Power Spectrum"=w1157:dynamicdata, "error out"=w1158:errorcluster)
                      }
                    }
                  }
                  frame 1 {
                    n143 = case shown="4" w1174 {
                      tunnel: w1173 -> [w1178 w1192 w1206 w1220 w1234 w1248 w1262 w1276 w1290 w1304]
                      tunnel: w1172 -> [w1177 w1191 w1205 w1219 w1233 w1247 w1261 w1275 w1289 w1303]
                      tunnel: [w1176 w1190 w1204 w1218 w1232 w1246 w1260 w1274 w1288 w1302] -> w1171
                      tunnel: [w1175 w1189 w1203 w1217 w1231 w1245 w1259 w1273 w1287 w1301] -> w1170
                      frame 0, Default {
                        n144 = xnode "Spectral Measurements"("Signals"=w1177, "error in (no error)"=w1178) -> ("Power Spectrum"=w1175:dynamicdata, "error out"=w1176:errorcluster)  [unwired: 1 in, 1 out]
                      }
                      frame 1 {
                        n145 = xnode "Spectral Measurements"("Signals"=w1191, "error in (no error)"=w1192) -> ("Power Spectrum"=w1189:dynamicdata, "error out"=w1190:errorcluster)  [unwired: 1 in, 1 out]
                      }
                      frame 2 {
                        n146 = xnode "Spectral Measurements"("Signals"=w1205, "error in (no error)"=w1206) -> ("Power Spectrum"=w1203:dynamicdata, "error out"=w1204:errorcluster)  [unwired: 1 in, 1 out]
                      }
                      frame 3 {
                        n147 = xnode "Spectral Measurements"("Signals"=w1219, "error in (no error)"=w1220) -> ("Power Spectrum"=w1217:dynamicdata, "error out"=w1218:errorcluster)  [unwired: 1 in, 1 out]
                      }
                      frame 4 {
                        n148 = xnode "Spectral Measurements"("Signals"=w1233, "error in (no error)"=w1234) -> ("Power Spectrum"=w1231:dynamicdata, "error out"=w1232:errorcluster)  [unwired: 1 in, 1 out]
                      }
                      frame 5 {
                        n149 = xnode "Spectral Measurements"("Signals"=w1247, "error in (no error)"=w1248) -> ("Power Spectrum"=w1245:dynamicdata, "error out"=w1246:errorcluster)  [unwired: 1 in, 1 out]
                      }
                      frame 6 {
                        n150 = xnode "Spectral Measurements"("Signals"=w1261, "error in (no error)"=w1262) -> ("Power Spectrum"=w1259:dynamicdata, "error out"=w1260:errorcluster)  [unwired: 1 in, 1 out]
                      }
                      frame 7 {
                        n151 = xnode "Spectral Measurements"("Signals"=w1275, "error in (no error)"=w1276) -> ("Power Spectrum"=w1273:dynamicdata, "error out"=w1274:errorcluster)  [unwired: 1 in, 1 out]
                      }
                      frame 8 {
                        n152 = xnode "Spectral Measurements"("Signals"=w1289, "error in (no error)"=w1290) -> ("Power Spectrum"=w1287:dynamicdata, "error out"=w1288:errorcluster)  [unwired: 1 in, 1 out]
                      }
                      frame 9 {
                        n153 = xnode "Spectral Measurements"("Signals"=w1303, "error in (no error)"=w1304) -> ("Power Spectrum"=w1301:dynamicdata, "error out"=w1302:errorcluster)  [unwired: 1 in, 1 out]
                      }
                    }
                  }
                  frame 2 {
                    n154 = case shown="8" w1319 {
                      tunnel: w1318 -> [w1323 w1337 w1351 w1365 w1379 w1393 w1407 w1421 w1435 w1449]
                      tunnel: w1317 -> [w1322 w1336 w1350 w1364 w1378 w1392 w1406 w1420 w1434 w1448]
                      tunnel: [w1321 w1335 w1349 w1363 w1377 w1391 w1405 w1419 w1433 w1447] -> w1316
                      tunnel: [w1320 w1334 w1348 w1362 w1376 w1390 w1404 w1418 w1432 w1446] -> w1315
                      frame 0, Default {
                        n155 = xnode "Spectral Measurements"("Signals"=w1322, "error in (no error)"=w1323) -> ("Power Spectrum"=w1320:dynamicdata, "error out"=w1321:errorcluster)  [unwired: 1 in, 1 out]
                      }
                      frame 1 {
                        n156 = xnode "Spectral Measurements"("Signals"=w1336, "error in (no error)"=w1337) -> ("Power Spectrum"=w1334:dynamicdata, "error out"=w1335:errorcluster)  [unwired: 1 in, 1 out]
                      }
                      frame 2 {
                        n157 = xnode "Spectral Measurements"("Signals"=w1350, "error in (no error)"=w1351) -> ("Power Spectrum"=w1348:dynamicdata, "error out"=w1349:errorcluster)  [unwired: 1 in, 1 out]
                      }
                      frame 3 {
                        n158 = xnode "Spectral Measurements"("Signals"=w1364, "error in (no error)"=w1365) -> ("Power Spectrum"=w1362:dynamicdata, "error out"=w1363:errorcluster)  [unwired: 1 in, 1 out]
                      }
                      frame 4 {
                        n159 = xnode "Spectral Measurements"("Signals"=w1378, "error in (no error)"=w1379) -> ("Power Spectrum"=w1376:dynamicdata, "error out"=w1377:errorcluster)  [unwired: 1 in, 1 out]
                      }
                      frame 5 {
                        n160 = xnode "Spectral Measurements"("Signals"=w1392, "error in (no error)"=w1393) -> ("Power Spectrum"=w1390:dynamicdata, "error out"=w1391:errorcluster)  [unwired: 1 in, 1 out]
                      }
                      frame 6 {
                        n161 = xnode "Spectral Measurements"("Signals"=w1406, "error in (no error)"=w1407) -> ("Power Spectrum"=w1404:dynamicdata, "error out"=w1405:errorcluster)  [unwired: 1 in, 1 out]
                      }
                      frame 7 {
                        n162 = xnode "Spectral Measurements"("Signals"=w1420, "error in (no error)"=w1421) -> ("Power Spectrum"=w1418:dynamicdata, "error out"=w1419:errorcluster)  [unwired: 1 in, 1 out]
                      }
                      frame 8 {
                        n163 = xnode "Spectral Measurements"("Signals"=w1434, "error in (no error)"=w1435) -> ("Power Spectrum"=w1432:dynamicdata, "error out"=w1433:errorcluster)  [unwired: 1 in, 1 out]
                      }
                      frame 9 {
                        n164 = xnode "Spectral Measurements"("Signals"=w1448, "error in (no error)"=w1449) -> ("Power Spectrum"=w1446:dynamicdata, "error out"=w1447:errorcluster)  [unwired: 1 in, 1 out]
                      }
                    }
                  }
                }
              }
              frame 3 {
                n165 = case shown="2" w1465 {
                  tunnel: w1464 -> [w1470 w1605 w1750]
                  tunnel: w1463 -> [w1469 w1604 w1749]
                  tunnel: w1462 -> [w1468 w1603 w1748]
                  tunnel: [w1467 w1602 w1747] -> w1461
                  tunnel: [w1466 w1601 w1746] -> w1460
                  frame 0, Default {
                    n166 = case shown="0, Default" w1470 {
                      tunnel: w1469 -> [w1474 w1487 w1500 w1513 w1526 w1539 w1552 w1565 w1578 w1591]
                      tunnel: w1468 -> [w1473 w1486 w1499 w1512 w1525 w1538 w1551 w1564 w1577 w1590]
                      tunnel: [w1472 w1485 w1498 w1511 w1524 w1537 w1550 w1563 w1576 w1589] -> w1467
                      tunnel: [w1471 w1484 w1497 w1510 w1523 w1536 w1549 w1562 w1575 w1588] -> w1466
                      frame 0, Default {
                        n167 = xnode "Spectral Measurements"("Signals"=w1473, "error in (no error)"=w1474) -> ("PSD"=w1471:dynamicdata, "error out"=w1472:errorcluster)
                      }
                      frame 1 {
                        n168 = xnode "Spectral Measurements"("Signals"=w1486, "error in (no error)"=w1487) -> ("PSD"=w1484:dynamicdata, "error out"=w1485:errorcluster)
                      }
                      frame 2 {
                        n169 = xnode "Spectral Measurements"("Signals"=w1499, "error in (no error)"=w1500) -> ("PSD"=w1497:dynamicdata, "error out"=w1498:errorcluster)
                      }
                      frame 3 {
                        n170 = xnode "Spectral Measurements"("Signals"=w1512, "error in (no error)"=w1513) -> ("PSD"=w1510:dynamicdata, "error out"=w1511:errorcluster)
                      }
                      frame 4 {
                        n171 = xnode "Spectral Measurements"("Signals"=w1525, "error in (no error)"=w1526) -> ("PSD"=w1523:dynamicdata, "error out"=w1524:errorcluster)
                      }
                      frame 5 {
                        n172 = xnode "Spectral Measurements"("Signals"=w1538, "error in (no error)"=w1539) -> ("PSD"=w1536:dynamicdata, "error out"=w1537:errorcluster)
                      }
                      frame 6 {
                        n173 = xnode "Spectral Measurements"("Signals"=w1551, "error in (no error)"=w1552) -> ("PSD"=w1549:dynamicdata, "error out"=w1550:errorcluster)
                      }
                      frame 7 {
                        n174 = xnode "Spectral Measurements"("Signals"=w1564, "error in (no error)"=w1565) -> ("PSD"=w1562:dynamicdata, "error out"=w1563:errorcluster)
                      }
                      frame 8 {
                        n175 = xnode "Spectral Measurements"("Signals"=w1577, "error in (no error)"=w1578) -> ("PSD"=w1575:dynamicdata, "error out"=w1576:errorcluster)
                      }
                      frame 9 {
                        n176 = xnode "Spectral Measurements"("Signals"=w1590, "error in (no error)"=w1591) -> ("PSD"=w1588:dynamicdata, "error out"=w1589:errorcluster)
                      }
                    }
                  }
                  frame 1 {
                    n177 = case shown="9" w1605 {
                      tunnel: w1604 -> [w1609 w1623 w1637 w1651 w1665 w1679 w1693 w1707 w1721 w1735]
                      tunnel: w1603 -> [w1608 w1622 w1636 w1650 w1664 w1678 w1692 w1706 w1720 w1734]
                      tunnel: [w1607 w1621 w1635 w1649 w1663 w1677 w1691 w1705 w1719 w1733] -> w1602
                      tunnel: [w1606 w1620 w1634 w1648 w1662 w1676 w1690 w1704 w1718 w1732] -> w1601
                      frame 0, Default {
                        n178 = xnode "Spectral Measurements"("Signals"=w1608, "error in (no error)"=w1609) -> ("PSD"=w1606:dynamicdata, "error out"=w1607:errorcluster)  [unwired: 1 in, 1 out]
                      }
                      frame 1 {
                        n179 = xnode "Spectral Measurements"("Signals"=w1622, "error in (no error)"=w1623) -> ("PSD"=w1620:dynamicdata, "error out"=w1621:errorcluster)  [unwired: 1 in, 1 out]
                      }
                      frame 2 {
                        n180 = xnode "Spectral Measurements"("Signals"=w1636, "error in (no error)"=w1637) -> ("PSD"=w1634:dynamicdata, "error out"=w1635:errorcluster)  [unwired: 1 in, 1 out]
                      }
                      frame 3 {
                        n181 = xnode "Spectral Measurements"("Signals"=w1650, "error in (no error)"=w1651) -> ("PSD"=w1648:dynamicdata, "error out"=w1649:errorcluster)  [unwired: 1 in, 1 out]
                      }
                      frame 4 {
                        n182 = xnode "Spectral Measurements"("Signals"=w1664, "error in (no error)"=w1665) -> ("PSD"=w1662:dynamicdata, "error out"=w1663:errorcluster)  [unwired: 1 in, 1 out]
                      }
                      frame 5 {
                        n183 = xnode "Spectral Measurements"("Signals"=w1678, "error in (no error)"=w1679) -> ("PSD"=w1676:dynamicdata, "error out"=w1677:errorcluster)  [unwired: 1 in, 1 out]
                      }
                      frame 6 {
                        n184 = xnode "Spectral Measurements"("Signals"=w1692, "error in (no error)"=w1693) -> ("PSD"=w1690:dynamicdata, "error out"=w1691:errorcluster)  [unwired: 1 in, 1 out]
                      }
                      frame 7 {
                        n185 = xnode "Spectral Measurements"("Signals"=w1706, "error in (no error)"=w1707) -> ("PSD"=w1704:dynamicdata, "error out"=w1705:errorcluster)  [unwired: 1 in, 1 out]
                      }
                      frame 8 {
                        n186 = xnode "Spectral Measurements"("Signals"=w1720, "error in (no error)"=w1721) -> ("PSD"=w1718:dynamicdata, "error out"=w1719:errorcluster)  [unwired: 1 in, 1 out]
                      }
                      frame 9 {
                        n187 = xnode "Spectral Measurements"("Signals"=w1734, "error in (no error)"=w1735) -> ("PSD"=w1732:dynamicdata, "error out"=w1733:errorcluster)  [unwired: 1 in, 1 out]
                      }
                    }
                  }
                  frame 2 {
                    n188 = case shown="9" w1750 {
                      tunnel: w1749 -> [w1754 w1768 w1782 w1796 w1810 w1824 w1838 w1852 w1866 w1880]
                      tunnel: w1748 -> [w1753 w1767 w1781 w1795 w1809 w1823 w1837 w1851 w1865 w1879]
                      tunnel: [w1752 w1766 w1780 w1794 w1808 w1822 w1836 w1850 w1864 w1878] -> w1747
                      tunnel: [w1751 w1765 w1779 w1793 w1807 w1821 w1835 w1849 w1863 w1877] -> w1746
                      frame 0, Default {
                        n189 = xnode "Spectral Measurements"("Signals"=w1753, "error in (no error)"=w1754) -> ("PSD"=w1751:dynamicdata, "error out"=w1752:errorcluster)  [unwired: 1 in, 1 out]
                      }
                      frame 1 {
                        n190 = xnode "Spectral Measurements"("Signals"=w1767, "error in (no error)"=w1768) -> ("PSD"=w1765:dynamicdata, "error out"=w1766:errorcluster)  [unwired: 1 in, 1 out]
                      }
                      frame 2 {
                        n191 = xnode "Spectral Measurements"("Signals"=w1781, "error in (no error)"=w1782) -> ("PSD"=w1779:dynamicdata, "error out"=w1780:errorcluster)  [unwired: 1 in, 1 out]
                      }
                      frame 3 {
                        n192 = xnode "Spectral Measurements"("Signals"=w1795, "error in (no error)"=w1796) -> ("PSD"=w1793:dynamicdata, "error out"=w1794:errorcluster)  [unwired: 1 in, 1 out]
                      }
                      frame 4 {
                        n193 = xnode "Spectral Measurements"("Signals"=w1809, "error in (no error)"=w1810) -> ("PSD"=w1807:dynamicdata, "error out"=w1808:errorcluster)  [unwired: 1 in, 1 out]
                      }
                      frame 5 {
                        n194 = xnode "Spectral Measurements"("Signals"=w1823, "error in (no error)"=w1824) -> ("PSD"=w1821:dynamicdata, "error out"=w1822:errorcluster)  [unwired: 1 in, 1 out]
                      }
                      frame 6 {
                        n195 = xnode "Spectral Measurements"("Signals"=w1837, "error in (no error)"=w1838) -> ("PSD"=w1835:dynamicdata, "error out"=w1836:errorcluster)  [unwired: 1 in, 1 out]
                      }
                      frame 7 {
                        n196 = xnode "Spectral Measurements"("Signals"=w1851, "error in (no error)"=w1852) -> ("PSD"=w1849:dynamicdata, "error out"=w1850:errorcluster)  [unwired: 1 in, 1 out]
                      }
                      frame 8 {
                        n197 = xnode "Spectral Measurements"("Signals"=w1865, "error in (no error)"=w1866) -> ("PSD"=w1863:dynamicdata, "error out"=w1864:errorcluster)  [unwired: 1 in, 1 out]
                      }
                      frame 9 {
                        n198 = xnode "Spectral Measurements"("Signals"=w1879, "error in (no error)"=w1880) -> ("PSD"=w1877:dynamicdata, "error out"=w1878:errorcluster)  [unwired: 1 in, 1 out]
                      }
                    }
                  }
                }
              }
            }
          }
        }
        "FFT Graph" <- w85
      }
    }
    n199 = Or(x=w15, y="?") -> (x .or. y?=w19:bool)
  }
  n200 = call <instrlib>:"niScope Close.vi"("instrument handle"=w3, "error in"=w5) -> ("error out"=w12:errorcluster)  [unwired: 13 in]
  n201 = call <vilib>:"Simple Error Handler.vi"("error in (no error)"=w12) -> ()  [unwired: 4 in, 5 out]
